vi "MotorControlRW.vi"(7 "timeout (msec)":u32=5000, 8 "error in (no error)":errorcluster, 9 "end":string=">>>", 10 "payload":string, 11 "VISA in":refnum<visa-resource-name>) -> (0 "error out":errorcluster, 1 "reply":string, 2 "rows":string[](array[string]), 3 "VISA Out":refnum<visa-resource-name>, 4 "Timed out":bool)   [LabVIEW 2022 SP3]
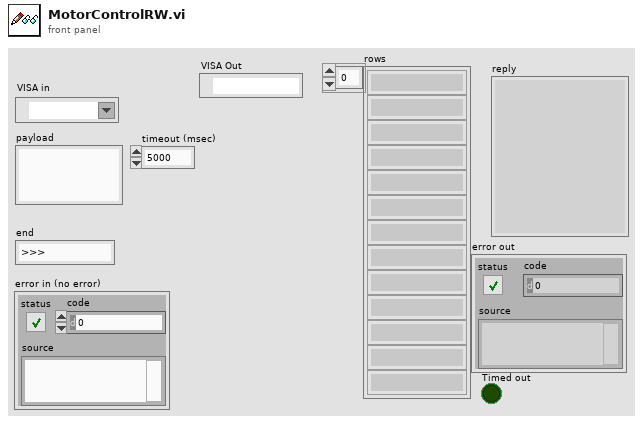
[diagram p1: front panel]
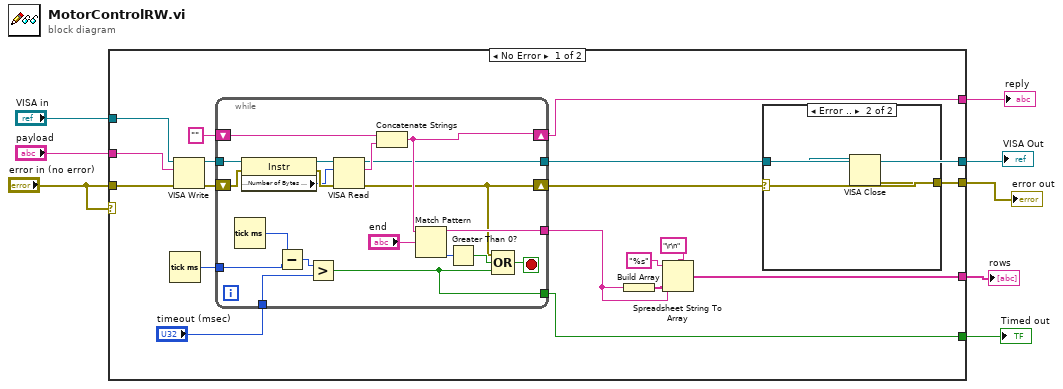
[diagram p0: block diagram]
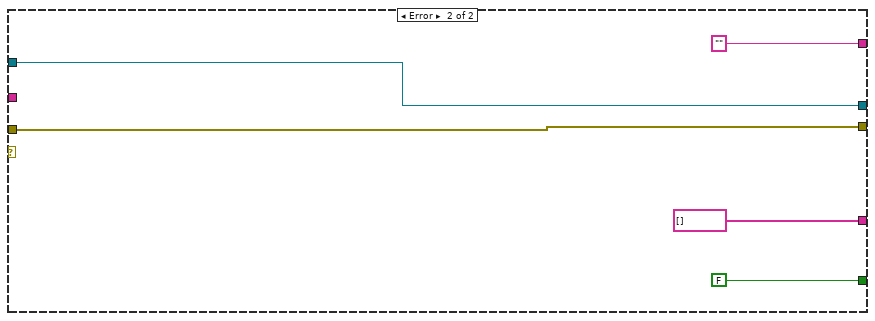
[diagram p3: hidden frame]
diagram:
  n1 = case shown="No Error" "error in (no error)" {
    tunnel: "payload" -> [w22 _]
    tunnel: "error in (no error)" -> [w21 w51]
    tunnel: "VISA in" -> [w9 w52]
    tunnel: [w15 ""] -> w5
    tunnel: [w14 w52] -> w4
    tunnel: [w10 string[] []] -> w3
    tunnel: [w13 FALSE] -> w2
    tunnel: [w12 w51] -> w1
    frame No Error {
      n2 = Tick Count (ms)() -> (millisecond timer value=w17:u32)
      n3 = VISA Write(VISA resource name=w9, write buffer=w22, error in (no error)=w21) -> (VISA resource name out=w24:refnum<visa-resource-name>, error out=w23:errorcluster)  [unwired: 1 out]
      n4 = while {
        tunnel: w24 -> [w47]
        shift-right: [w43] -> w15
        shift-left: "" -> [w45]
        tunnel: [w40] -> w11
        shift-right: [w28] -> w12
        shift-left: w23 -> [w39]
        tunnel: w17 -> [w35]
        tunnel: [w31] -> w13
        tunnel: [w30] -> w14
        tunnel: "timeout (msec)" -> [w29]
        stop <- w32 stop-if-true
        n5 = Tick Count (ms)() -> (millisecond timer value=w36:u32)
        n6 = property class="Instr"(reference=w47, error in=w39) -> (reference out=w46:refnum<visa-resource-name>, error out=w38:errorcluster, "Serial Settings:Number of Bytes at Serial Port"=w37:u32)
        n7 = Subtract(x=w36, y=w35) -> (x-y=w34:u32)
        n8 = Greater?(x=w34, y=w29) -> (0:w31:bool)
        n9 = VISA Read(VISA resource name=w46, byte count=w37, error in (no error)=w38) -> (VISA resource name out=w30:refnum<visa-resource-name>, read buffer=w44:string, error out=w28:errorcluster)  [unwired: 1 out]
        n10 = Concatenate Strings(w45, w44) -> (w43:string)
        n11 = Match Pattern(string=w43, regular expression="end") -> (before substring=w40:string, offset past match=w41:i32)  [unwired: 1 in, 2 out]
        n12 = Greater Than 0?(x=w41) -> (x > 0?=w33:bool)
        n13 = Compound Arithmetic op=OR(w28, w33, w31) -> (w32:bool)
      }
      n14 = Build Array(w11) -> (w20:string[])
      n15 = Spreadsheet String To Array(delimiter (Tab)="\r\n", format string="%s", spreadsheet string=w11, array type (2D Dbl)=w20) -> (array=w10:string[])
      n16 = case shown="Error .." w12 {
        tunnel: [_ w27] -> _
        tunnel: w14 -> [_ w26]
        frame No Error {
        }
        frame Error {
          n17 = VISA Close(VISA resource name=w26) -> (error out=w27:errorcluster)  [unwired: 1 in]
        }
      }
    }
    frame Error {
    }
  }
  "reply" <- w5
  "VISA Out" <- w4
  "rows" <- w3
  "Timed out" <- w2
  "error out" <- w1
